vi "Initialize Pod.vi"() -> (0 "error out":errorcluster, 2 "Telemetry Queue":refnum<queue>)   [LabVIEW 2017]
uses:
  Type Defs/telemetryReading.ctl
  Type Defs/PodState.ctl
  <vilib>/myRIO/Instrument Drivers/Onboard IO/DIO/typedefs/DIO Reference.ctl
  <vilib>/myRIO/Common/Instrument Driver Framework/Utilities/typedefs/myRIO Generic Hardware Reference.ctl
  <vilib>/myRIO/Common/Instrument Driver Framework/Utilities/typedefs/Hardware Version Enum.ctl
  <vilib>/myRIO/Common/Instrument Driver Framework/Utilities/typedefs/myRIO v1.0 Reference.ctl
  <vilib>/myRIO/Common/Instrument Driver Framework/Utilities/typedefs/Generic FPGA Reference.ctl
  <vilib>/myRIO/Common/Instrument Driver Framework/myRIO v1.0/DIO/typedefs/DIO Channels List.ctl
  <vilib>/myRIO/Common/Instrument Driver Framework/myRIO v1.0/DIO/typedefs/DIO Channels Enum.ctl
  <vilib>/userdefined/High Color/nirio_resource_hc.ctl
  <vilib>/myRIO/Common/Instrument Driver Framework/Utilities/vis/Is FPGA Ref Available.vi
  <vilib>/myRIO/Common/Instrument Driver Framework/myRIO v1.0/DIO/vis/myRIO v1.1 Open DIO.vi
  <vilib>/myRIO/Instrument Drivers/Onboard IO/DIO/vis/Write.vi
  <vilib>/myRIO/Common/Instrument Driver Framework/Utilities/vis/Validate Channels.vi
  <vilib>/myRIO/Common/Instrument Driver Framework/myRIO v1.0/DIO/vis/myRIO v1.0 Reserve DIO.vi
  <vilib>/myRIO/Common/Instrument Driver Framework/myRIO v1.0/Resource Manager/vis/myRIO v1.0 Reserve Channel List.vi
  <vilib>/myRIO/Common/Instrument Driver Framework/myRIO v1.0/DIO/vis/myRIO v1.0 Build MUX Configuration DIO.vi
  <vilib>/myRIO/Common/Instrument Driver Framework/myRIO v1.0/Resource Manager/vis/myRIO v1.0 Reserve Channel.vi
  <vilib>/myRIO/Common/Instrument Driver Framework/myRIO v1.0/Resource Manager/vis/myRIO v1.0 Unreserve Channel.vi
  <vilib>/myRIO/Common/Instrument Driver Framework/myRIO v1.0/Resource Manager/vis/myRIO v1.0 Create Configuration List.vi
  <vilib>/myRIO/Common/Instrument Driver Framework/myRIO v1.0/Resource Manager/vis/myRIO v1.0 Build Mutex Name.vi
  <vilib>/Utility/VariantDataType/GetNumericInfo.vi
  <vilib>/Utility/error.llb/Error Cluster From Error Code.vi
  <vilib>/myRIO/Common/Instrument Driver Framework/myRIO v1.0/myRIO v1.1 Open.vi
  <vilib>/myRIO/Common/Instrument Driver Framework/Utilities/vis/IO Manager.vi
  <vilib>/myRIO/Common/Instrument Driver Framework/Utilities/vis/Configuration Manager.vi
  <vilib>/myRIO/Common/Instrument Driver Framework/myRIO v1.0/Resource Manager/vis/myRIO v1.0 Configure IO.vi
  <vilib>/myRIO/Common/Instrument Driver Framework/myRIO v1.0/myRIO v1.0 Close.vi
  <vilib>/myRIO/Common/Instrument Driver Framework/myRIO v1.0/DIO/vis/myRIO v1.0 Write DIO.vi
  <vilib>/myRIO/Express VI/Onboard Devices/LED/LED Express VI.xnode
  <vilib>/myRIO/Instrument Drivers/Onboard IO/DIO/vis/myRIO DIO Open.xnode
  <vilib>/myRIO/Instrument Drivers/Onboard IO/DIO/DIO.lvlib
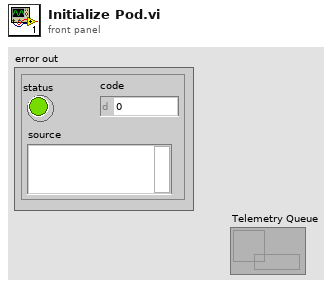
[diagram p1: front panel]
types:
  T1 = typedef "PodState.ctl" = enum16{"Initializing", "Pre-flight Testing", "Ready", "Pushing", "Coast", "Braking", "Pod-Stop", "Fault"}
  T2 = typedef "telemetryReading.ctl" = cluster{"Sensor:Reading":string, "Data":variant, "Time Stamp":timestamp}
  T3 = typedef "DIO.lvlib/DIO Reference.ctl" = cluster{"myRIO Reference":T4, "DIO Channels List":T8}
  T4 = typedef "myRIO Generic Hardware Reference.ctl" = cluster{"myRIO Model":T5, "myRIO Hardware Reference":T6}
  T5 = typedef "Hardware Version Enum.ctl" = enum16{"Unknown", "myRIO-1900", "myRIO-1950", "roboRIO", "NI ELVIS RIO CM"}
  T6 = typedef "myRIO v1.0 Reference.ctl" = cluster{"Generic FPGA Reference":T7, "Allow multiple opens":bool}
  T7 = typedef "Generic FPGA Reference.ctl" = refnum<k20>
  T8 = typedef "DIO Channels List.ctl" = T9[]
  T9 = typedef "DIO Channels Enum.ctl" = enum16{"Not Connected", "C/DIO0", "C/DIO1", "C/DIO2", "C/DIO3", "C/DIO4", "C/DIO5", "C/DIO6", "C/DIO7", "A/DIO0", "A/DIO1", "A/DIO2", "A/DIO3", "A/DIO4", "A/DIO5", "A/DIO6", "A/DIO7", "A/DIO8", "A/DIO9", "A/DIO10", "A/DIO11", "A/DIO12", "A/DIO13", "A/DIO14", "A/DIO15", "B/DIO0", "B/DIO1", "B/DIO2", "B/DIO3", "B/DIO4", "B/DIO5", "B/DIO6", "B/DIO7", "B/DIO8", "B/DIO9", "B/DIO10", "B/DIO11", "B/DIO12", "B/DIO13", "B/DIO14", "B/DIO15", "LED0", "LED1", "LED2", "LED3", "Button0", "DIO/DIO0", "DIO/DIO1", "DIO/DIO2", "DIO/DIO3", "DIO/DIO4", "DIO/DIO5", "DIO/DIO6", "DIO/DIO7", "DIO/DIO8", "DIO/DIO9", "SPI/CS0", "SPI/CS1", "SPI/CS2", "SPI/CS3", "LED RADIO (Green)", "LED RADIO (Red)", "LED COMM (Green)", "LED COMM (Red)", "LED MODE (Green)", "LED MODE (Red)"}
  T10 = typedef "nirio_resource_hc.ctl" = tag
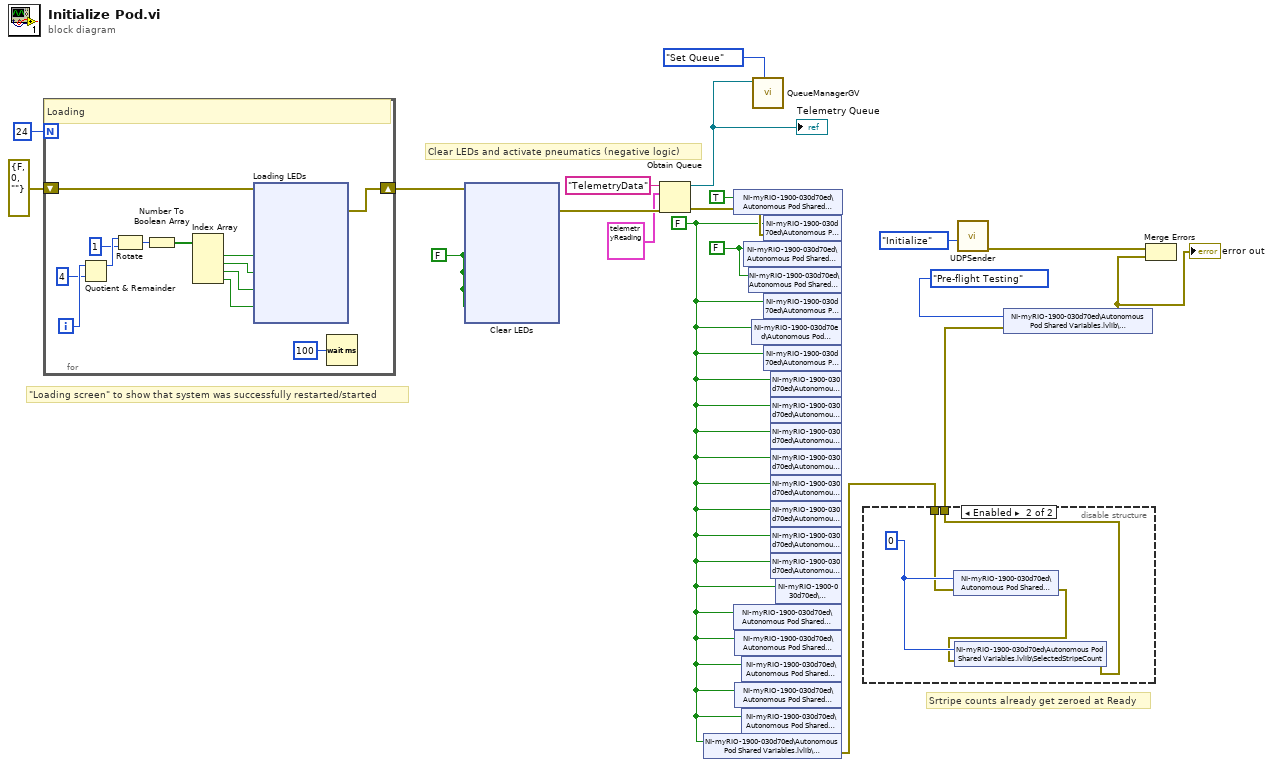
[diagram p0: block diagram]
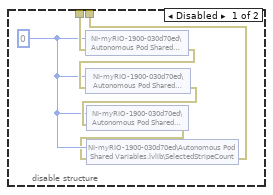
[diagram p2: hidden frame]
diagram:
  w8 = FALSE ("sendNcData")
  w4 = FALSE ("sendNcData")
  w40 = FALSE ("Levitation")
  # "Srtripe counts already get zeroed at Ready"
  # "Clear LEDs and activate pneumatics (negative logic)"
  # "\"Loading screen\" to show that system was successfully restarted/started"
  n1 = for {
    N: 24 -> [_]
    shift-right: [w48] -> w39
    shift-left: errorcluster {"status"=FALSE, "code"=0, "source"=""} ("error out") -> [w47]
    i -> [w53]
    # "Loading"
    n2 = Quotient & Remainder(x=w53, y=4) -> (x-y*floor(x/y)=w46:i32)  [unwired: 1 out]
    n3 = Rotate(1:i16 1 ("y"), 2:w46) -> (0:w50:i16)
    n4 = Number To Boolean Array(number=w50) -> (Boolean array=w49:bool[])
    n5 = Index Array(array=w49) -> (element #1=w44:bool, element #2=w41:bool, element #3=w42:bool, element #4=w43:bool)  [unwired: 4 in]
    n6 = xnode "Loading LEDs"("LED0"=w44, "LED1"=w41, "LED2"=w42, "LED3"=w43, "error in (no error)"=w47) -> ("error out"=w48:errorcluster)
    n7 = Wait (ms)(milliseconds to wait=u32 100) -> ()  [unwired: 1 out]
  }
  n8 = xnode "Clear LEDs"("LED0"=w40, "LED1"=w40, "LED2"=w40, "LED3"=w40, "error in (no error)"=w39) -> ("error out"=w36:errorcluster)
  n9 = Obtain Queue(name (unnamed)="TelemetryData", element data type=T2 {"Sensor:Reading"="", "Data"=variant, "Time Stamp"=timestamp(3584563538.456057 s since 1904-01-01)} ("Telemetry Reading"), error in (no error)=w36) -> (queue out=w33:refnum<queue>, error out=w29:errorcluster)  [unwired: 2 in, 1 out]
  "Telemetry Queue" <- w33
  n10 = shared-variable "NI-myRIO-1900-030d70ed\\Autonomous Pod Shared Variables.lvlib\\sendNcData"(TRUE ("sendNcData"), error in=w29) -> (error out=w9:errorcluster)
  n11 = call "QueueManagerGV.vi"("Command"=enum16{"Get", "Set Logging", "Set Queue"}."Set Queue", "Queue in"=w33) -> ()  [unwired: 8 in, 2 out]
  n12 = shared-variable "NI-myRIO-1900-030d70ed\\Autonomous Pod Shared Variables.lvlib\\2way1"(w4, error in=w9) -> (error out=w28:errorcluster)
  n13 = shared-variable "NI-myRIO-1900-030d70ed\\Autonomous Pod Shared Variables.lvlib\\MagBrake"(w8, error in=w28) -> (error out=w27:errorcluster)
  n14 = shared-variable "NI-myRIO-1900-030d70ed\\Autonomous Pod Shared Variables.lvlib\\FricBrake"(w8, error in=w27) -> (error out=w26:errorcluster)
  n15 = shared-variable "NI-myRIO-1900-030d70ed\\Autonomous Pod Shared Variables.lvlib\\2way2"(w4, error in=w26) -> (error out=w25:errorcluster)
  n16 = shared-variable "NI-myRIO-1900-030d70ed\\Autonomous Pod Shared Variables.lvlib\\PneuAct"(w4, error in=w25) -> (error out=w24:errorcluster)
  n17 = shared-variable "NI-myRIO-1900-030d70ed\\Autonomous Pod Shared Variables.lvlib\\2way3"(w4, error in=w24) -> (error out=w23:errorcluster)
  n18 = shared-variable "NI-myRIO-1900-030d70ed\\Autonomous Pod Shared Variables.lvlib\\ToF1"(w4, error in=w23) -> (error out=w22:errorcluster)
  n19 = shared-variable "NI-myRIO-1900-030d70ed\\Autonomous Pod Shared Variables.lvlib\\ToF2"(w4, error in=w22) -> (error out=w21:errorcluster)
  n20 = shared-variable "NI-myRIO-1900-030d70ed\\Autonomous Pod Shared Variables.lvlib\\ToF3"(w4, error in=w21) -> (error out=w20:errorcluster)
  n21 = shared-variable "NI-myRIO-1900-030d70ed\\Autonomous Pod Shared Variables.lvlib\\ToF4"(w4, error in=w20) -> (error out=w19:errorcluster)
  n22 = shared-variable "NI-myRIO-1900-030d70ed\\Autonomous Pod Shared Variables.lvlib\\ToF5"(w4, error in=w19) -> (error out=w18:errorcluster)
  n23 = shared-variable "NI-myRIO-1900-030d70ed\\Autonomous Pod Shared Variables.lvlib\\ToF6"(w4, error in=w18) -> (error out=w17:errorcluster)
  n24 = shared-variable "NI-myRIO-1900-030d70ed\\Autonomous Pod Shared Variables.lvlib\\ToF7"(w4, error in=w17) -> (error out=w16:errorcluster)
  n25 = shared-variable "NI-myRIO-1900-030d70ed\\Autonomous Pod Shared Variables.lvlib\\ToF8"(w4, error in=w16) -> (error out=w15:errorcluster)
  n26 = shared-variable "NI-myRIO-1900-030d70ed\\Autonomous Pod Shared Variables.lvlib\\Cap"(w4, error in=w15) -> (error out=w14:errorcluster)
  n27 = shared-variable "NI-myRIO-1900-030d70ed\\Autonomous Pod Shared Variables.lvlib\\SensePower"(w4, error in=w14) -> (error out=w13:errorcluster)
  n28 = shared-variable "NI-myRIO-1900-030d70ed\\Autonomous Pod Shared Variables.lvlib\\3way1Open"(w4, error in=w13) -> (error out=w12:errorcluster)
  n29 = shared-variable "NI-myRIO-1900-030d70ed\\Autonomous Pod Shared Variables.lvlib\\3way1Port"(w4, error in=w12) -> (error out=w11:errorcluster)
  n30 = shared-variable "NI-myRIO-1900-030d70ed\\Autonomous Pod Shared Variables.lvlib\\3way2Open"(w4, error in=w11) -> (error out=w10:errorcluster)
  n31 = shared-variable "NI-myRIO-1900-030d70ed\\Autonomous Pod Shared Variables.lvlib\\3way2Port"(w4, error in=w10) -> (error out=w3:errorcluster)
  n32 = shared-variable "NI-myRIO-1900-030d70ed\\Autonomous Pod Shared Variables.lvlib\\AutoSequenceOn"(w4, error in=w3) -> (error out=w2:errorcluster)
  n33 = disable-structure shown="Enabled" {
    disable-tunnel: w2 -> [w95 w100]
    disable-tunnel: [w92 w98] -> w1
    frame Disabled {
      w94 = u32 0 ("TimerValue")
      n34 = shared-variable "NI-myRIO-1900-030d70ed\\Autonomous Pod Shared Variables.lvlib\\TimerLimit"(w94, error in=w95) -> (error out=w97:errorcluster)
      n35 = shared-variable "NI-myRIO-1900-030d70ed\\Autonomous Pod Shared Variables.lvlib\\TimerValue"(w94, error in=w97) -> (error out=w96:errorcluster)
      n36 = shared-variable "NI-myRIO-1900-030d70ed\\Autonomous Pod Shared Variables.lvlib\\StripeLimit"(w94, error in=w96) -> (error out=w93:errorcluster)
      n37 = shared-variable "NI-myRIO-1900-030d70ed\\Autonomous Pod Shared Variables.lvlib\\SelectedStripeCount"(w94, error in=w93) -> (error out=w92:errorcluster)
    }
    frame Enabled {
      w101 = u32 0 ("TimerValue")
      n38 = shared-variable "NI-myRIO-1900-030d70ed\\Autonomous Pod Shared Variables.lvlib\\TimerValue"(w101, error in=w100) -> (error out=w99:errorcluster)
      n39 = shared-variable "NI-myRIO-1900-030d70ed\\Autonomous Pod Shared Variables.lvlib\\SelectedStripeCount"(w101, error in=w99) -> (error out=w98:errorcluster)
    }
  }
  n40 = call "UDPSender.vi"("Action"=enum16{"Send", "Initialize", "Close"}."Initialize") -> ("error out"=w7:errorcluster)  [unwired: 10 in]
  n41 = shared-variable "NI-myRIO-1900-030d70ed\\Autonomous Pod Shared Variables.lvlib\\PodStateCommand"(PodState."Pre-flight Testing" ("PodState"), error in=w1) -> (error out=w5:errorcluster)
  "error out" <- w5
  n42 = Merge Errors(w7, w5) -> ()  [unwired: 1 out]
